vi "ClosePreprocSessionAndDeleteFile.vi"(8 "error in (no error)":errorcluster, 11 "Python.lvclass":refnum<class "Python.lvclass">) -> (0 "error out":errorcluster, 3 "Python.lvclass":refnum<class "Python.lvclass">)   [LabVIEW 2020, in "Python.lvclass"]
uses:
  Python.lvclass
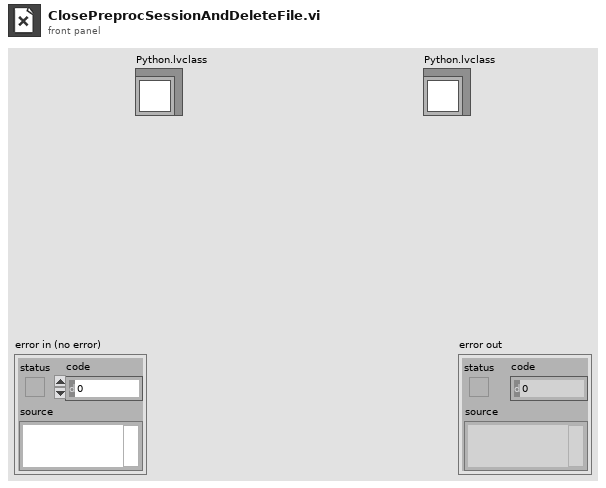
[diagram p1: front panel]
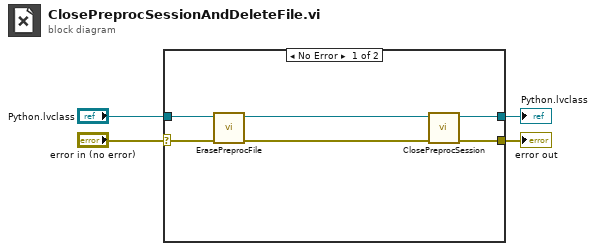
[diagram p0: block diagram]
diagram:
  n1 = case shown="No Error" "error in (no error)" {
    selector: "error in (no error)" -> [w7 w12]
    tunnel: [w5 w12] -> w3
    tunnel: [w8 w11] -> w1
    tunnel: "Python.lvclass" -> [w10 w11]
    frame No Error {
      n2 = call-dynamic "ErasePreprocFile.vi"("error in (no error)"=w7, "Python in"=w10) -> ("error out"=w6:errorcluster, "Python out"=w9:refnum<class "Python.lvclass">)  [unwired: 8 in]
      n3 = call-dynamic "ClosePreprocSession.vi"("error in (no error)"=w6, "Python in"=w9) -> ("error out"=w5:errorcluster, "Python out"=w8:refnum<class "Python.lvclass">)  [unwired: 8 in]
    }
    frame Error {
    }
  }
  "error out" <- w3
  "Python.lvclass" <- w1
